vi "Stop Analog Output.vi"(8 "error in (no error)":errorcluster, 10 "AO Task ID's In":u32[](array[numeric])) -> (0 "error out":errorcluster)   [LabVIEW 2009]
uses:
  Acquisition Settings.vi
  <vilib>/Daq/1easyio.llb/AO Update Channels (scaled array).vi
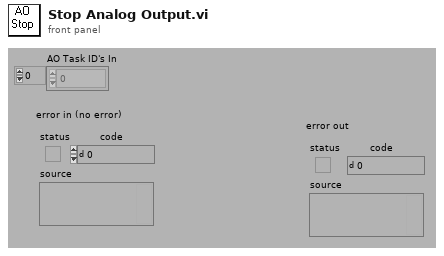
[diagram p1: front panel]
types:
  T1 = cluster{"device":i16, "channel":tag, "buffer size":i32, "Signal Description":cluster{"Name":string, "signal type":enum16{"Sine Wave", "Square Wave", "Sawtooth", "Triangle Wave"}, "period":dbl, "amplitude":dbl, "phase (0 deg)":dbl, "offset (0.0)":dbl, "resting voltage":dbl, "% duty cycle":dbl}[], "clock source (internal:1)":u16, "Clock Line Number":i16}[]
  T2 = cluster{"Name":string, "signal type":enum16{"Sine Wave", "Square Wave", "Sawtooth", "Triangle Wave"}, "period":dbl, "amplitude":dbl, "phase (0 deg)":dbl, "offset (0.0)":dbl, "resting voltage":dbl, "% duty cycle":dbl}[]
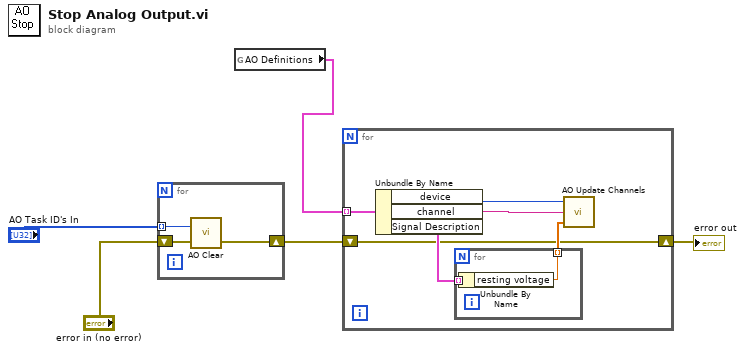
[diagram p0: block diagram]
diagram:
  n1 = for {
    tunnel: "AO Task ID's In" -> [w8] mode=indexing
    shift-right: [w6] -> w3
    shift-left: "error in (no error)" -> [w7]
    n2 = call <vilib>:"AO Clear.vi"("error in (no error)"=w7, "taskID in"=w8) -> ("error out"=w6:errorcluster)  [unwired: 4 in, 1 out]
  }
  n3 = global read "Acquisition Settings.vi" "AO Definitions"() -> (w1:T1)
  n4 = for {
    shift-right: [w9] -> w2
    shift-left: w3 -> [w9]
    tunnel: w1 -> [w14] mode=indexing
    n5 = Unbundle By Name(w14) -> ("device"=w10:i16, "channel"=w11:tag, "Signal Description"=w13:T2)
    n6 = for {
      tunnel: w13 -> [w16] mode=indexing
      tunnel: [w15] -> w12 mode=indexing
      n7 = Unbundle By Name(w16) -> ("resting voltage"=w15:dbl)
    }
    n8 = call-poly <vilib>:"AO Update Channels.vi"("values"=w12, "channels (0)"=w11, "device"=w10) -> ()
  }
  "error out" <- w2
